vi "RTE Test Result Path and File Names.vi"(8 "error in (no error)":errorcluster) -> (0 "error out":errorcluster, 1 "PPL Test_Strings.txt":string, 2 "PPL Test_Status.txt":string, 3 "HDH\\ProjectBuilder\\temp path":path)   [LabVIEW 2019, in "ProjectBuilder.lvlib" / "PPL Class Test.lvclass"]
uses:
  PPL Class Test.lvclass
  ProjectBuilder.lvlib
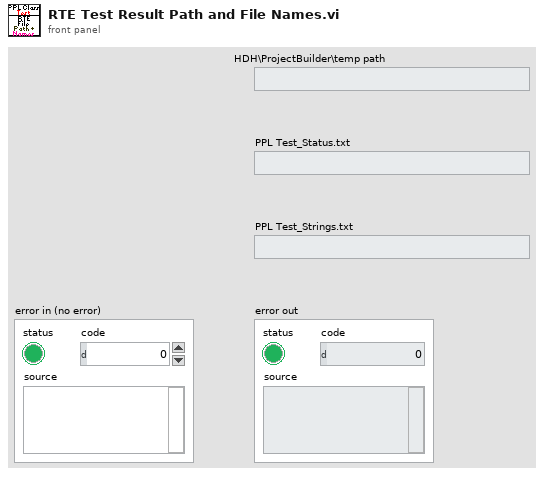
[diagram p1: front panel]
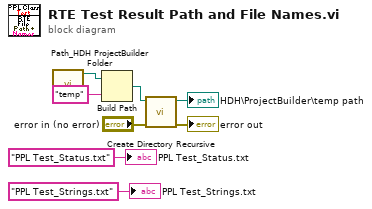
[diagram p0: block diagram]
diagram:
  n1 = call "Path_HDH ProjectBuilder Folder.vi"() -> ("HDH\\ProjectBuilder path"=w1:path)  [unwired: 11 in]
  n2 = Build Path(base path=w1, name or relative path="temp") -> (appended path=w3:path)
  n3 = call <vilib>:"Create Directory Recursive.vi"("error in (no error)"="error in (no error)", "directory"=w3) -> ("error out"=→"error out":errorcluster, "directory copy"=→"HDH\\ProjectBuilder\\temp path":path)  [unwired: 3 in, 1 out]
  "PPL Test_Strings.txt" <- "PPL Test_Strings.txt"
  "PPL Test_Status.txt" <- "PPL Test_Status.txt"
